vi "ADI_IMU_ADIS16448_Get Angles.vi"(8 "error in":errorcluster, 11 "ADI IMU DevRef":T1={"DevStatus"={"status"=FALSE, "code"=0, "source"=""}, "Handle"=27, "SPI Bus"=enum."SPI MXP", "Device Found"=TRUE, "Device Ready"=FALSE, "Yaw Axis"=enum."Z", "AHRS Algorithm"=enum."Complementary", "Serial"=118, "Lot ID 2"=5379, "Lot ID 1"=118, "Bytes Per Sample"=0, "Calibrate On Open?"=FALSE}) -> (0 "error out":errorcluster, 1 "Sensor Ready Out":bool, 2 "IMU Angles Out":T3, 3 "ADI IMU DevRef Out":T1={"DevStatus"={"status"=FALSE, "code"=0, "source"=""}, "Handle"=27, "SPI Bus"=enum."SPI MXP", "Device Found"=TRUE, "Device Ready"=FALSE, "Yaw Axis"=enum."Z", "AHRS Algorithm"=enum."Complementary", "Serial"=118, "Lot ID 2"=5379, "Lot ID 1"=118, "Bytes Per Sample"=0, "Calibrate On Open?"=FALSE})   [LabVIEW 2018, in "ADIS16448_IMU.lvlib"]
doc: "Read accumulated angles from the Analog Devices IMU MXP board. Requires the IMU_Loop VI to be running in Periodic Tasks."
uses:
  ADIS16448_IMU.lvlib
  ADI_IMU_ADIS16448_IMUDevRef.ctl
  <vilib>/Rock Robotics/SystemInterfaces/spilib/spi_bus.ctl
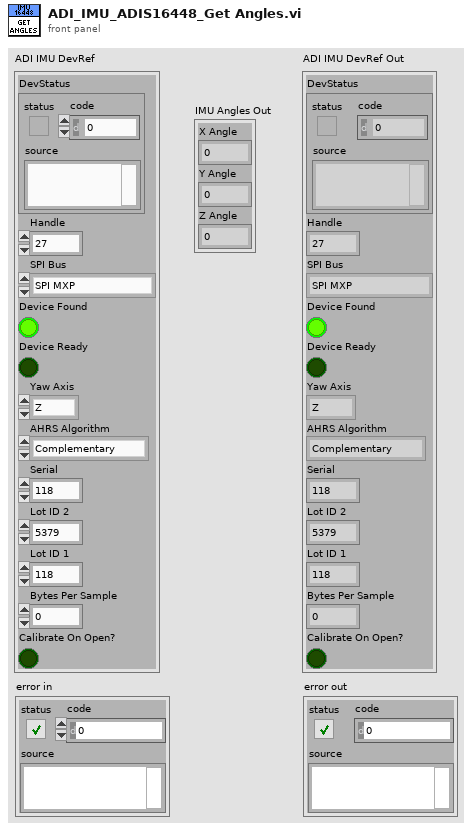
[diagram p1: front panel]
types:
  T1 = typedef "ADIS16448_IMU.lvlib/ADI_IMU_ADIS16448_IMUDevRef.ctl" = cluster{"DevStatus":errorcluster, "Handle":i32, "SPI Bus":T2, "Device Found":bool, "Device Ready":bool, "Yaw Axis":enum16{"X", "Y", "Z"}, "AHRS Algorithm":enum16{"Complementary", "Madgwick"}, "Serial":u16, "Lot ID 2":u16, "Lot ID 1":u16, "Bytes Per Sample":u16, "Calibrate On Open?":bool}
  T2 = typedef "spi_bus.ctl" = enum16{"SPI On-Board, CS0", "SPI On-Board, CS1", "SPI On-Board, CS2", "SPI On-Board, CS3", "SPI MXP", "Invalid"}
  T3 = cluster{"X Angle":dbl, "Y Angle":dbl, "Z Angle":dbl}
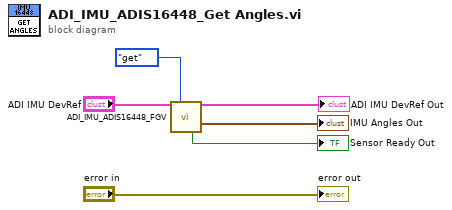
[diagram p0: block diagram]
diagram:
  n1 = call "ADI_IMU_ADIS16448_FGV.vi"("ADI IMU DevRef"="ADI IMU DevRef", "Operation"=enum16{"set", "get"}."get") -> ("ADI IMU DevRef Out"=→"ADI IMU DevRef Out":T1, "IMU Angles Out"=→"IMU Angles Out":T3, "Sensor Ready Out"=→"Sensor Ready Out":bool)  [unwired: 7 in, 4 out]
  "error out" <- "error in"
